vi "RC steering motor interpolation.vi"(11 "Value Channel 0":i32) -> (2 "Numeric":sgl, 3 "Boolean":bool)   [LabVIEW 2016]
doc: "Input\nValue Channel 0\n\nOutput\nSwitch direction\nDuty Cycle in\n\nInterpolates the value from channel 0 and determines if we going left or right and with what duty cycle."
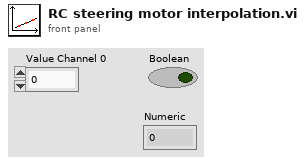
[diagram p1: front panel]
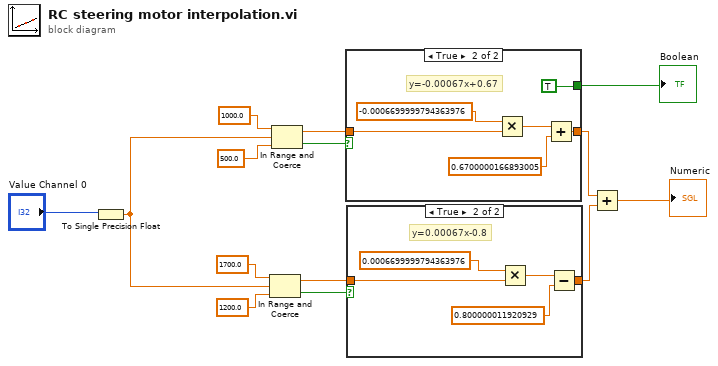
[diagram p0: block diagram]
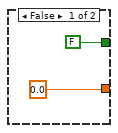
[diagram p2: hidden frame]
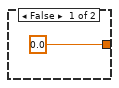
[diagram p3: hidden frame]
diagram:
  n1 = To Single Precision Float(number="Value Channel 0") -> (single precision float=w6:sgl)
  n2 = In Range and Coerce(upper limit=sgl 1700.0, x=w6, lower limit=sgl 1200.0) -> (coerced(x)=w7:sgl, In Range?=w10:bool)
  n3 = In Range and Coerce(upper limit=sgl 1000.0, x=w6, lower limit=sgl 500.0) -> (coerced(x)=w8:sgl, In Range?=w9:bool)
  n4 = case shown="True" w9 {
    tunnel: w8 -> [_ w19]
    tunnel: [sgl 0.0 w18] -> w11
    tunnel: [FALSE TRUE] -> w14
    frame False {
    }
    frame True {
      # "y=-0.00067x+0.67"
      n5 = Multiply(x=sgl -0.00067, y=w19) -> (x*y=w21:sgl)
      n6 = Add(x=w21, y=sgl 0.67) -> (x+y=w18:sgl)
    }
  }
  "Boolean" <- w14
  n7 = case shown="True" w10 {
    tunnel: w7 -> [_ w25]
    tunnel: [sgl 0.0 w24] -> w12
    frame False {
    }
    frame True {
      # "y=0.00067x-0.8"
      n8 = Multiply(x=sgl 0.00067, y=w25) -> (x*y=w27:sgl)
      n9 = Subtract(x=w27, y=sgl 0.8) -> (x-y=w24:sgl)
    }
  }
  n10 = Add(x=w11, y=w12) -> (x+y=→"Numeric":sgl)
